vi "Inst.Krohn-Hite-7008.AppLauncher.vi"(8 "error in":errorcluster, 10 "Config Window":bool, 11 "Debug Mode":bool) -> (0 "error out":errorcluster)   [LabVIEW 2019, in "Inst.KH7008.lvlib" / "Inst.Krohn-Hite-7008.lvclass"]
uses:
  Inst.Krohn-Hite-7008.lvclass
  <vilib>/JKI/JKI SMO/SMO/SMO.lvclass
  <vilib>/JKI/JKI SMO/SMO/Typedefs/SMOState --Enum.ctl
  <vilib>/JKI/JKI SMO/SMO.UI/SMO.UI.lvclass
  <userlib>/LevyLab/Instrument Framework/Instrument UI/Instrument UI.lvclass
  Inst UI.Krohn-Hite-7008/Inst UI.Krohn-Hite-7008.lvclass
  <userlib>/LevyLab/Instrument Framework/Instrument/Instrument.lvclass
  C:/Program Files/National Instruments/LabVIEW 2019/vi.lib/JKI/JKI SMO/SMO/SMO.lvclass
  C:/Program Files/National Instruments/LabVIEW 2019/vi.lib/JKI/JKI SMO/SMO.UI/SMO.UI.lvclass
  C:/Program Files/National Instruments/LabVIEW 2019/user.lib/LevyLab/Instrument Framework/Instrument Types/Amplifier/Instrument.Amplifier.lvclass
  C:/Program Files/National Instruments/LabVIEW 2019/user.lib/LevyLab/Instrument Framework/Instrument/Instrument.lvclass
  C:/Program Files/National Instruments/LabVIEW 2019/user.lib/LevyLab/Instrument Framework/Instrument UI/Instrument UI.lvclass
panel:
  in  "Examine Configuration.ini":bool
  in  "Splash Status":string="Push Start to Start..." caption="String"
  in  "Start Application":bool caption="Play"
  in  "Stop Application":bool caption="Stop"
  out "UI SMO State":T1=enum."Stopped"
  out "SMO State":T1
  # "Example Instrument SMO Test Launcher"
  # "For instructions on how to use the JKI State Machine Objects, examples and video tutorials, visit:\nhttp://jki.net/state-machine-objects/\n\nJKI State Machine Objects™\nhttp://jki.net/state-machine-objects/\nCopyright (C) 2005-2015, JKI <info@jki.net>\nALL RIGHTS RESERVED"
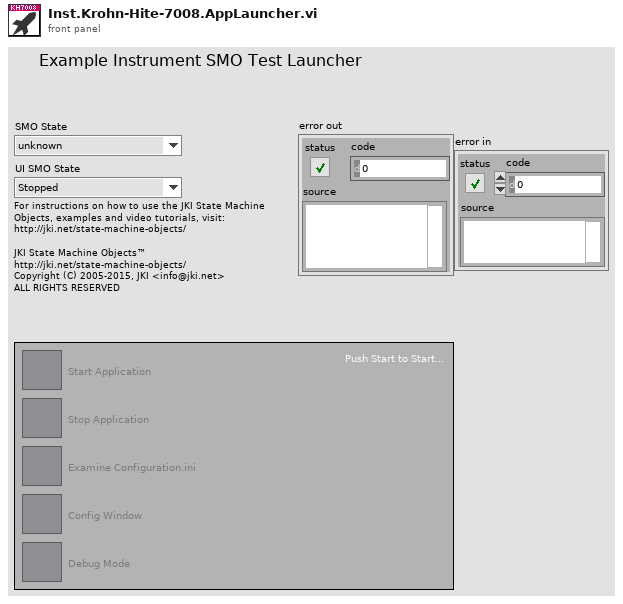
[diagram p1: front panel]
types:
  T1 = typedef "smo.lvlib/SMO.lvclass/SMOState --Enum.ctl" = enum16{"unknown", "Created", "Started", "Stopped"}
  T2 = enum32{"Invalid", "Standard", "Closed", "Hidden", "Minimized", "Maximized"}
  T3 = enum32{"invalid app kind", "Development System", "Run Time System", "Student Edition", "Embedded LabVIEW", "Evaluation", "Custom"}
  T4 = cluster{"Core":cluster{"Current VI Reference":refnum<vi>, "Close Panel on Exit?":bool}, "Instrument":refnum<class "Instrument.lvclass">, "Instrument UI":refnum<class "Instrument UI.lvclass">}
  T5 = cluster{"Current VI Reference":refnum<vi>, "Close Panel on Exit?":bool}
  T6 = typedef "smo.lvlib/SMO.lvclass/Public Events.ctl" = cluster{"Error":refnum<user-event>, "State":refnum<user-event>, "Reserve State":refnum<user-event>}
  T7 = cluster{"Event Registration Refnum":refnum<event-registration>, "Event Registration Refnum":refnum<event-registration>}
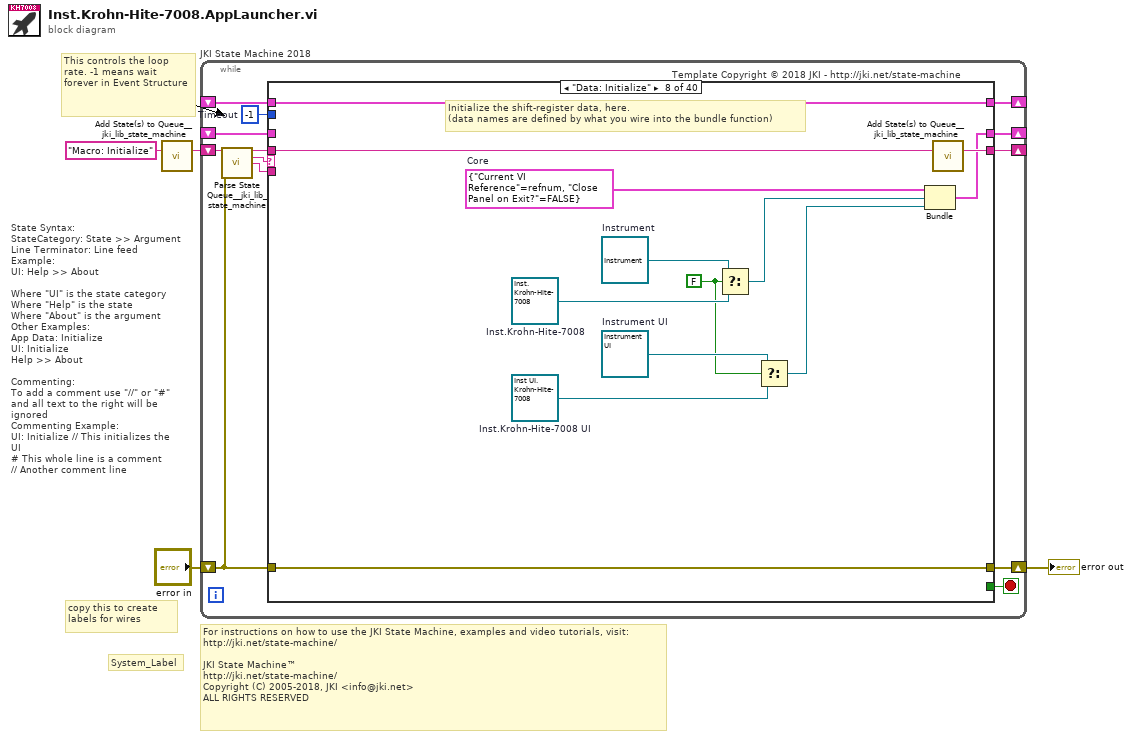
[diagram p0: block diagram]
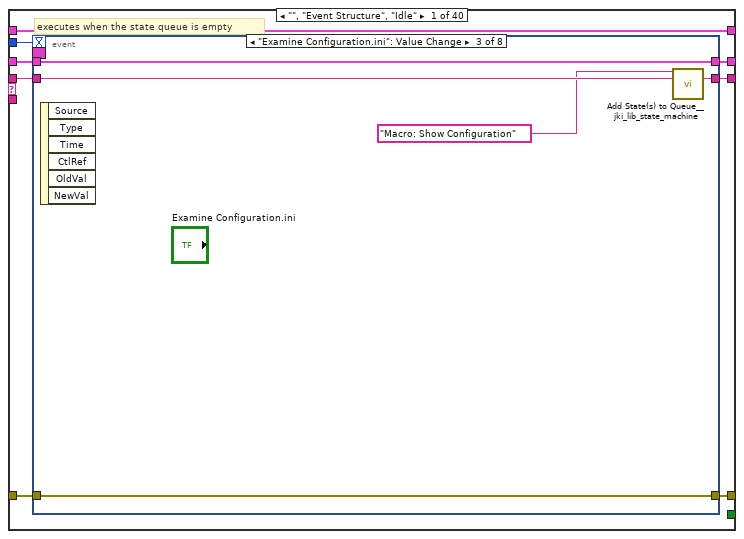
[diagram p2: hidden frame]
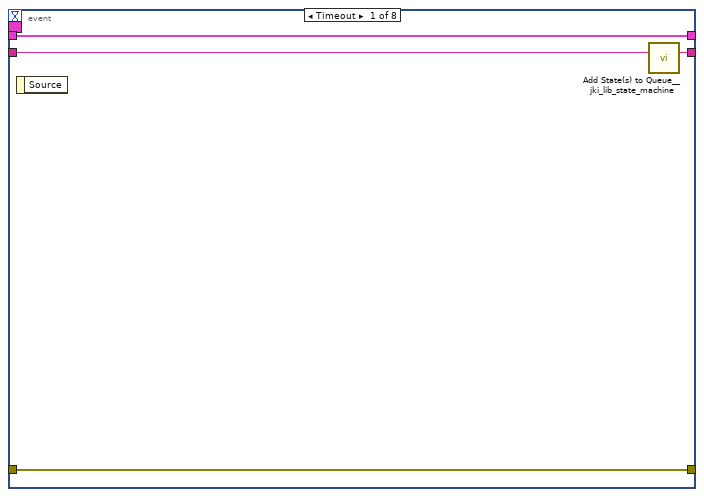
[diagram p3: hidden frame]
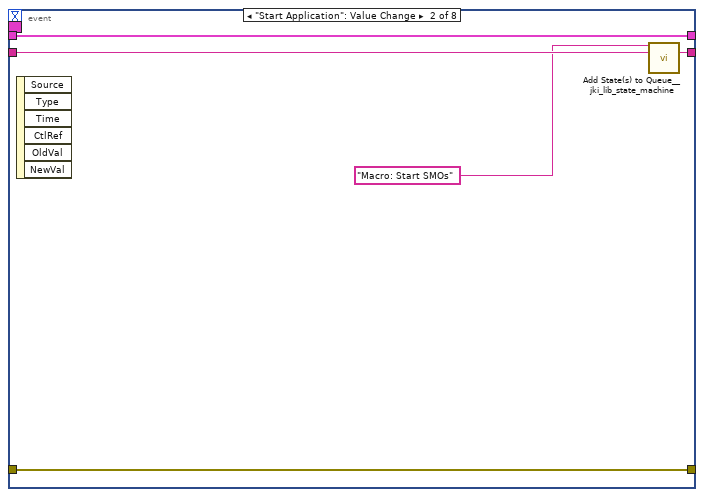
[diagram p4: hidden frame]
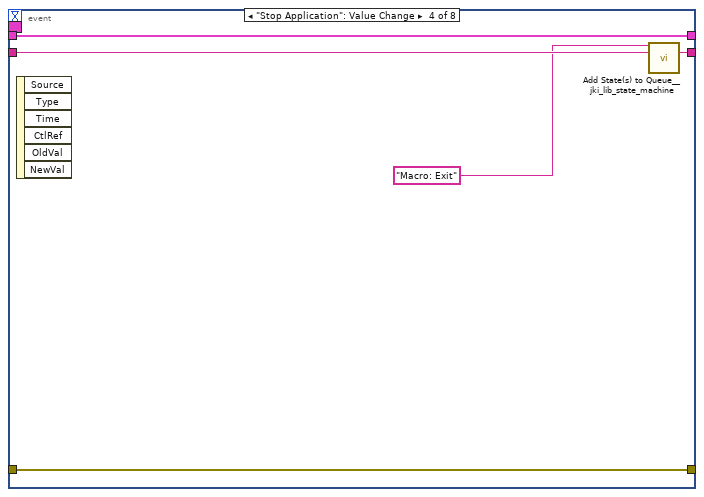
[diagram p5: hidden frame]
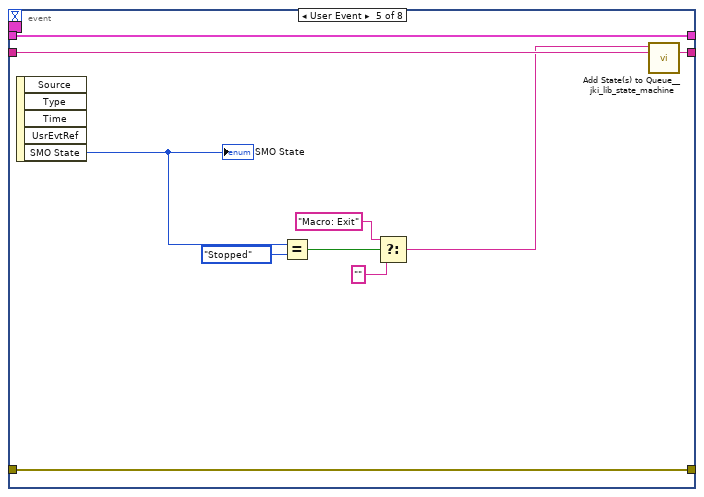
[diagram p6: hidden frame]
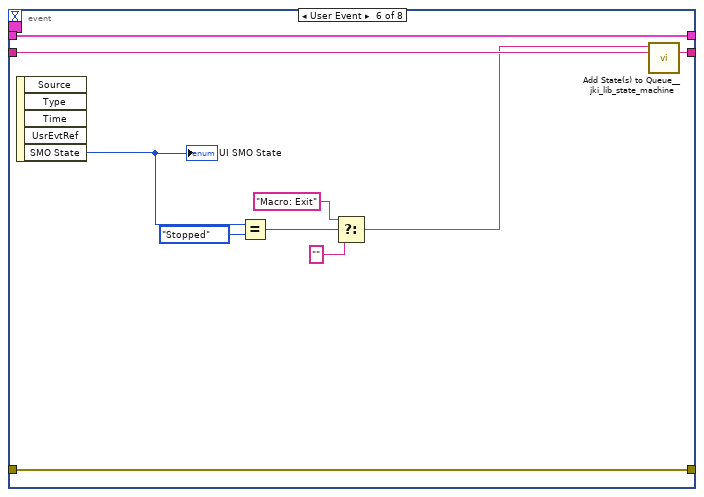
[diagram p7: hidden frame]
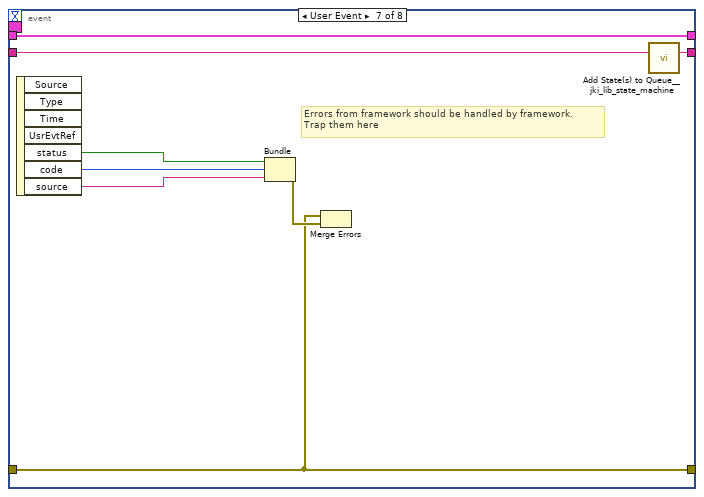
[diagram p8: hidden frame]
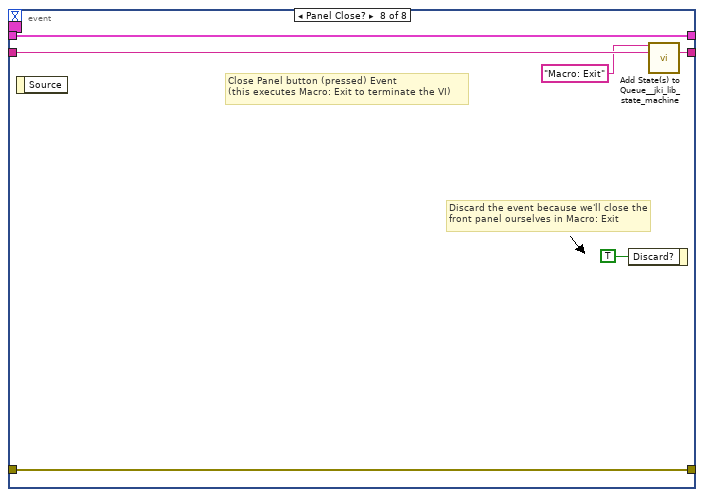
[diagram p9: hidden frame]
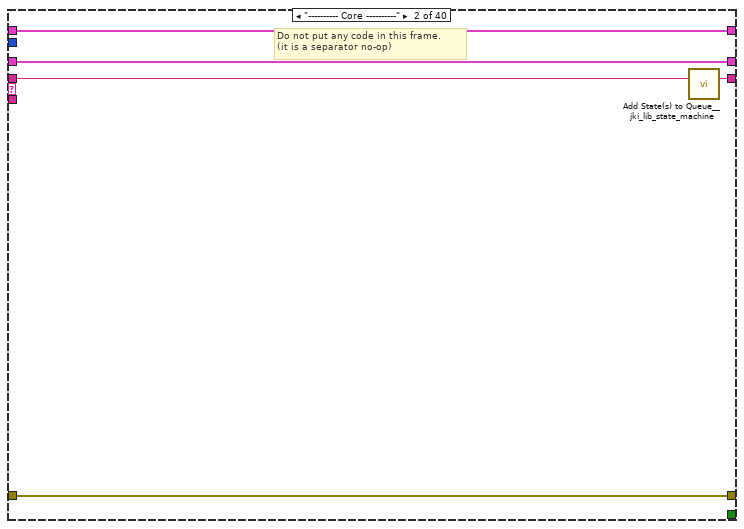
[diagram p10: hidden frame]
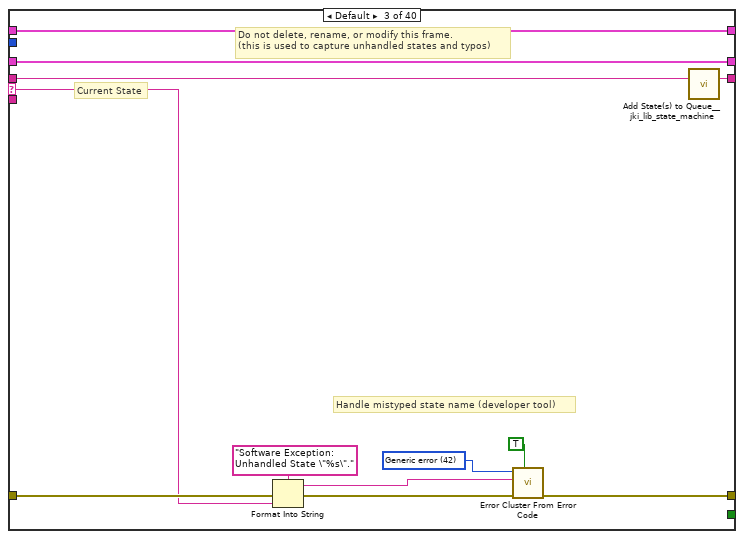
[diagram p11: hidden frame]
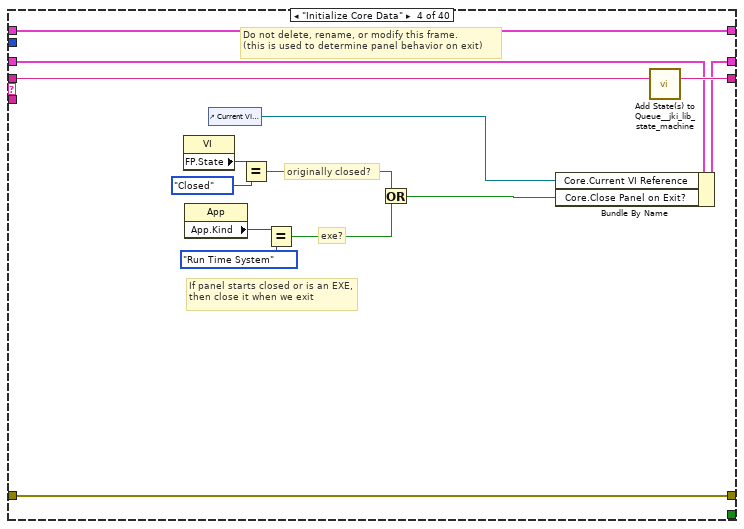
[diagram p12: hidden frame]
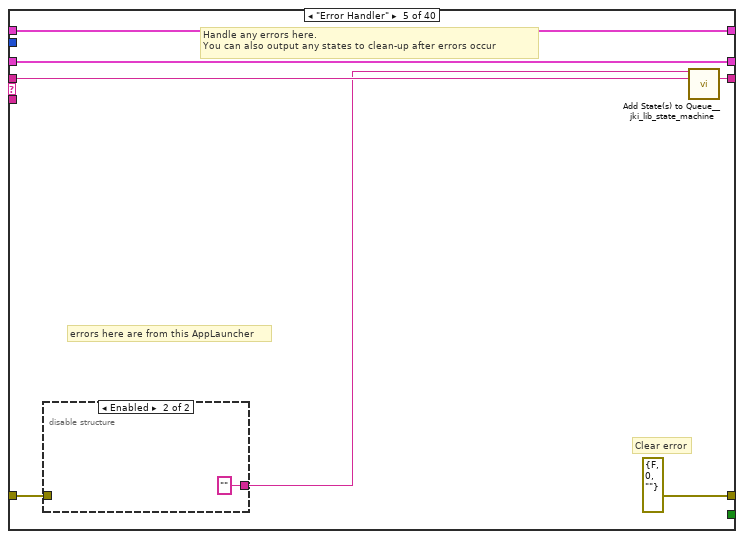
[diagram p13: hidden frame]
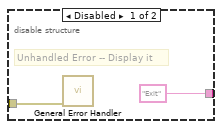
[diagram p14: hidden frame]
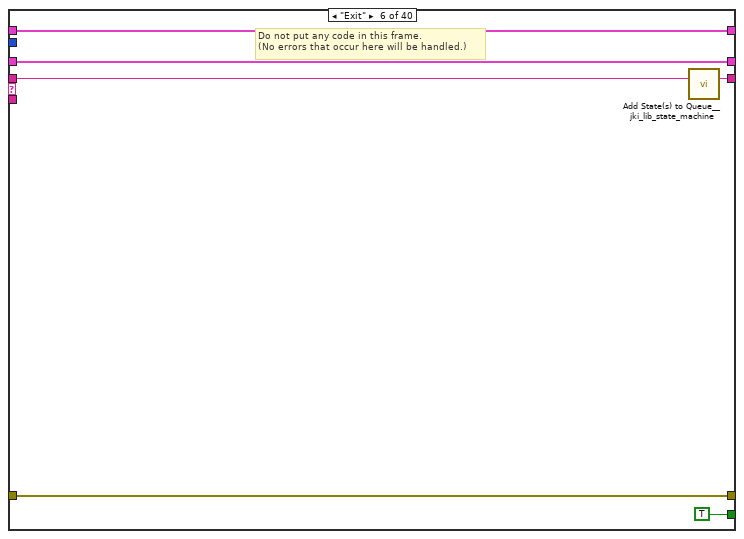
[diagram p15: hidden frame]
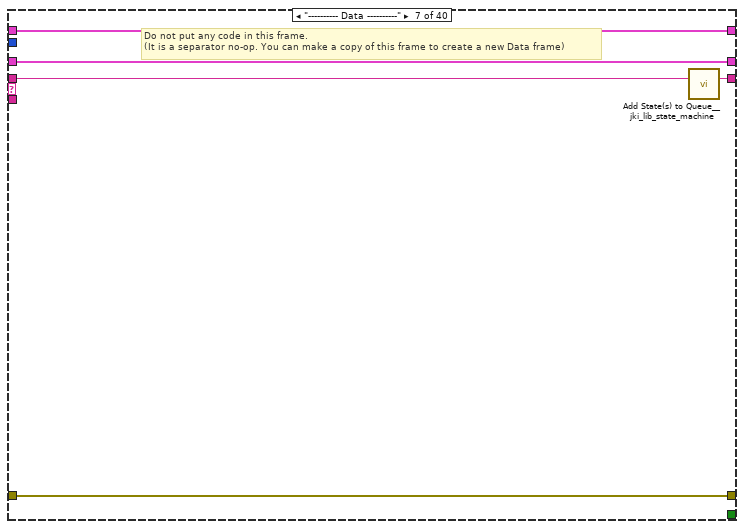
[diagram p16: hidden frame]
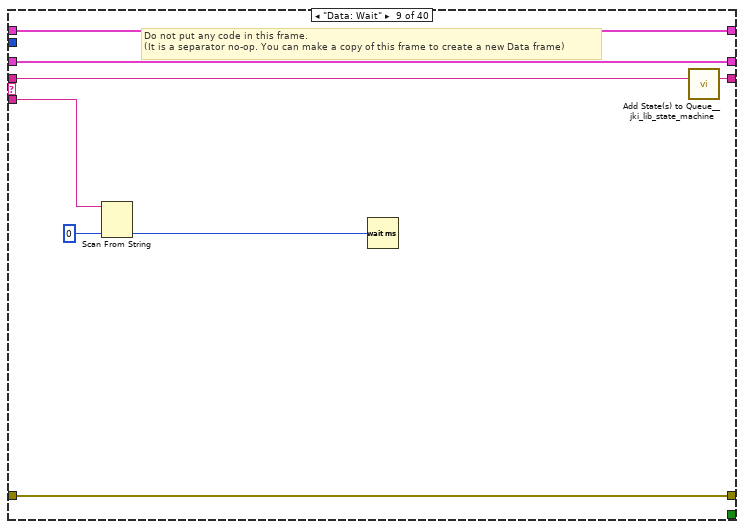
[diagram p17: hidden frame]
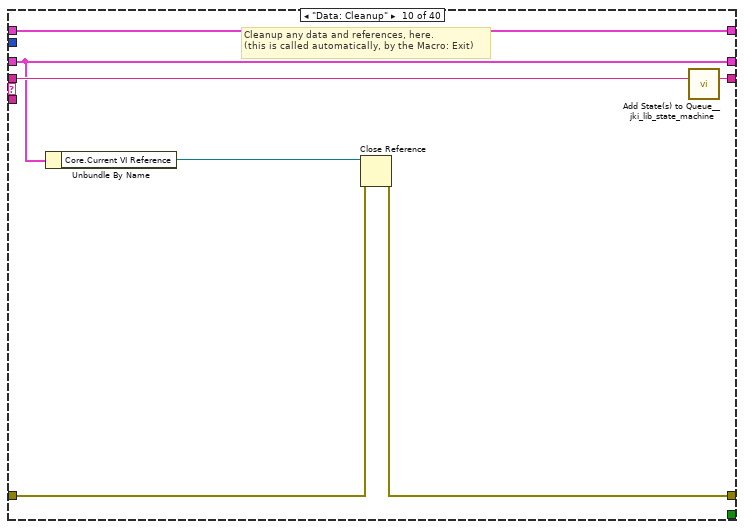
[diagram p18: hidden frame]
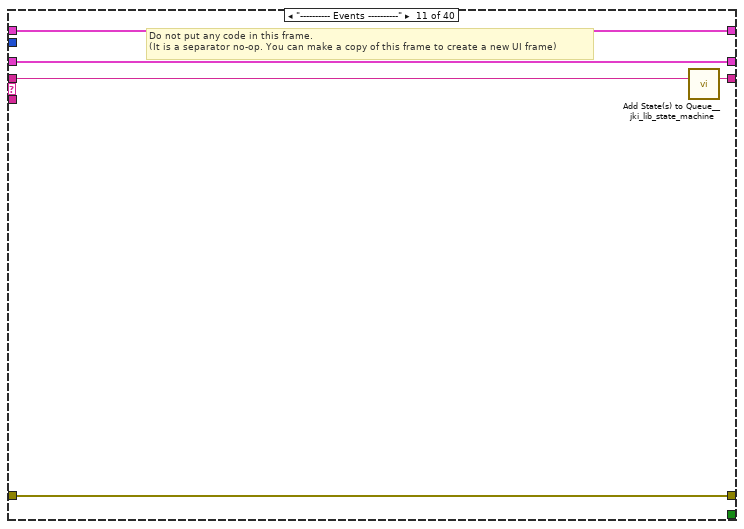
[diagram p19: hidden frame]
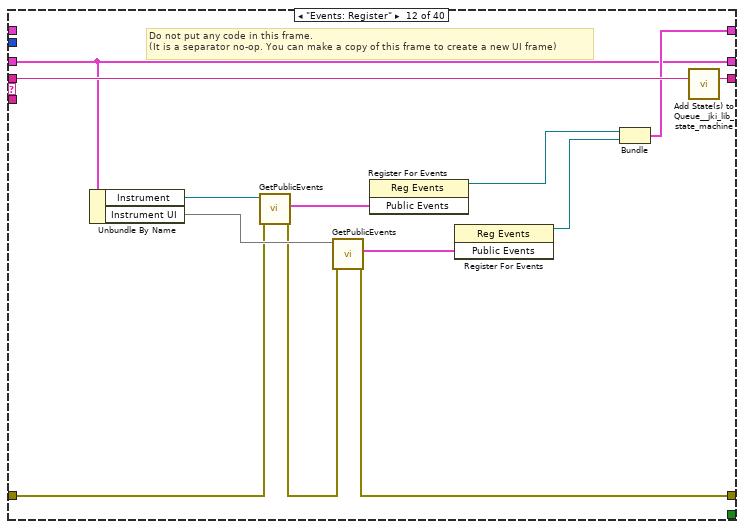
[diagram p20: hidden frame]
diagram:
  # "For instructions on how to use the JKI State Machine, examples and video tutorials, visit:\nhttp://jki.net/state-machine/\n\nJKI State Machine™\nhttp://jki.net/state-machine/\nCopyright (C) 2005-2018, JKI <info@jki.net>\nALL RIGHTS RESERVED"
  # "State Syntax:\nStateCategory: State >> Argument\nLine Terminator: Line feed\nExample:\nUI: Help >> About\n\nWhere \"UI\" is the state category\nWhere \"Help\" is the state\nWhere \"About\" is the argument\nOther Examples:\nApp Data: Initialize\nUI: Initialize\nHelp >> About\n\nCommenting:\nTo add a comment use \"//\" or \"#\" and all text to the right will be ignored\nCommenting Example:\nUI: Initialize // This initializes the UI\n# This whole line is a comment\n// Another comment line"
  # "copy this to create labels for wires"
  # "This controls the loop rate. -1 means wait forever in Event Structure"
  # "System_Label"
  n1 = call <vilib>:"Add State(s) to Queue__jki_lib_state_machine.vi"("State(s) in (\"\")"="Macro: Initialize") -> ("States Out"=w4:string)  [unwired: 14 in]
  n2 = while "JKI State Machine 2018" {
    shift-right: [w11] -> _
    shift-left: _ -> [w6]
    shift-right: [w14] -> w2
    shift-left: "error in" -> [w9]
    shift-right: [w13] -> _
    shift-left: w4 -> [w15]
    shift-right: [w8] -> _
    shift-left: _ -> [w7]
    stop <- w12 stop-if-true
    w10 = -1  # Timeout
    # "Template Copyright © 2018 JKI - http://jki.net/state-machine"
    n3 = call <vilib>:"Parse State Queue__jki_lib_state_machine.vi"("State Queue"=w15, "Error In (no error)"=w9) -> ("Remaining States"=w17:string, "Current State"=w5:string, "Arguments"=w16:string)  [unwired: 11 in]
    n4 = case shown="\"Data: Initialize\"" w5 {
      selector: w5 -> [_ _ w85 _ _ _ _ _ _ _ _ _ _ _ _ _ _ _ _ _ _ _ _ _ _ _ _ _ _ _ _ _ _ _ _ _ _ _ _ _]
      tunnel: w17 -> [w25 w83 w89 w109 w116 w125 w130 w143 w151 w158 w163 w176 w182 w187 w194 w201 w213 w291 w298 w303 w308 w314 w320 w326 w332 w344 w349 w360 w369 w379 w386 w397 w412 w427 w442 w457 w472 w481 w488 w493]
      tunnel: w16 -> [_ _ _ _ _ _ _ _ w146 _ _ _ _ _ _ w196 w207 _ _ _ _ _ _ _ _ _ _ _ _ _ _ _ _ _ _ _ _ _ w485 _]
      tunnel: [w22 w81 w91 w106 errorcluster {"status"=FALSE, "code"=0, "source"=""} ("error out") w122 w128 w138 w149 w154 w161 w165 w177 w185 w189 w197 w210 w281 w295 w301 w306 w312 w318 w324 w330 w342 w347 w356 w361 w370 w380 w393 w408 w423 w439 w454 w469 w479 w483 w491] -> w14
      tunnel: w9 -> [w21 w81 w90 w106 w112 w122 w128 w138 w149 w155 w161 w167 w178 w185 w191 w198 w211 w282 w292 w301 w306 w312 w318 w324 w330 w342 w347 w357 w362 w371 w381 w390 w404 w420 w437 w452 w465 w479 w484 w491]
      tunnel: [w24 w82 w88 w108 w115 w124 w129 w142 w150 w157 w162 w175 w181 w186 w193 w200 w212 w290 w297 w302 w307 w313 w319 w325 w331 w343 w348 w359 w368 w378 w385 w396 w411 w426 w441 w456 w471 w480 w487 w492] -> w13
      tunnel: [_ _ _ _ _ TRUE _ _ _ _ _ _ _ _ _ _ _ _ _ _ _ _ _ _ _ _ _ _ _ _ _ _ _ _ _ _ _ _ _ _] -> w12
      tunnel: [w20 w80 w87 w107 w113 w123 w127 w141 w148 w153 w160 w170 w180 w184 w192 w199 w209 w279 w294 w300 w305 w311 w317 w323 w329 w341 w346 w355 w364 w375 w383 w394 w409 w424 w438 w453 w468 w478 w486 w490] -> w11
      tunnel: w10 -> [w19 _ _ _ _ _ _ _ _ _ _ _ _ _ _ _ _ _ _ _ _ _ _ _ _ _ _ _ _ _ _ _ _ _ _ _ _ _ _ _]
      tunnel: [w18 w79 w84 w96 w111 w120 w126 w139 w147 w152 w159 w173 w179 w183 w190 w195 w206 w280 w296 w299 w304 w309 w315 w322 w328 w335 w345 w358 w367 w377 w384 w395 w410 w425 w440 w455 w470 w477 w482 w489] -> w8
      tunnel: w7 -> [w18 w79 w84 w96 w111 w120 w126 w139 w147 w152 w159 _ w179 w183 w190 w195 w206 w280 w296 w299 w304 w309 w315 w322 w328 w335 w345 w358 w367 w377 w384 w395 w410 w425 w440 w455 w470 w477 w482 w489]
      tunnel: w6 -> [w23 w80 w87 w102 w113 w123 w127 _ w148 w153 w160 w170 w180 w184 w192 w199 w209 w279 w294 w300 w305 w311 w317 w323 w329 w341 w346 w353 w365 w376 w383 w394 w409 w424 w438 w453 w468 w478 w486 w490]
      frame "", "Event Structure", "Idle" {
        # "executes when the state queue is empty"
        n5 = event shown="[2] \"Examine Configuration.ini\": Value Change" {
          selector: w18 -> [_ _ _ _ _ _ _ _]
          dyn-events: _ -> [_ _ _ _ _ _ _ _]
          timeout: w19 -> [_ _ _ _ _ _ _ _]
          tunnel: w25 -> [w29 w34 w39 w44 w54 w64 w72 w78]
          tunnel: [w28 w33 w38 w43 w53 w63 w71 w77] -> w24
          tunnel: w23 -> [w26 w31 w36 w41 w51 w61 w70 w75]
          tunnel: [w27 w32 w37 w42 w52 w62 w65 w76] -> w22
          tunnel: w21 -> [w27 w32 w37 w42 w52 w62 w65 w76]
          tunnel: [w26 w31 w36 w41 w51 w61 w70 w75] -> w20
          event Timeout {
            n6 = event-data() -> ()  [unwired: 1 in, 1 out]
            n7 = call <vilib>:"Add State(s) to Queue__jki_lib_state_machine.vi"("State(s) in (\"\")"=w29) -> ("States Out"=w28:string)  [unwired: 14 in]
          }
          event "Start Application": Value Change {
            n8 = event-data() -> ()  [unwired: 1 in, 6 out]
            n9 = call <vilib>:"Add State(s) to Queue__jki_lib_state_machine.vi"("State(s) in Front (\"\")"="Macro: Start SMOs" ("State(s) in Front (\"\")"), "State(s) in (\"\")"=w34) -> ("States Out"=w33:string)  [unwired: 13 in]
          }
          event "Examine Configuration.ini": Value Change {
            n10 = event-data() -> ()  [unwired: 1 in, 6 out]
            n11 = call <vilib>:"Add State(s) to Queue__jki_lib_state_machine.vi"("State(s) in Front (\"\")"="Macro: Show Configuration" ("State(s) in Front (\"\")"), "State(s) in (\"\")"=w39) -> ("States Out"=w38:string)  [unwired: 13 in]
          }
          event "Stop Application": Value Change {
            n12 = event-data() -> ()  [unwired: 1 in, 6 out]
            n13 = call <vilib>:"Add State(s) to Queue__jki_lib_state_machine.vi"("State(s) in Front (\"\")"="Macro: Exit" ("State(s) in Front (\"\")"), "State(s) in (\"\")"=w44) -> ("States Out"=w43:string)  [unwired: 13 in]
          }
          event User Event {
            n14 = event-data() -> ("SMO State"=w46:T1)  [unwired: 1 in, 4 out]
            "SMO State" <- w46
            n15 = Equal?(x=w46, y=SMOState_--Enum."Stopped") -> (x = y?=w49:bool)
            n16 = Select(t="Macro: Exit", s=w49, f="" ("State(s) in Front (\"\")")) -> (s? t:f=w45:string)
            n17 = call <vilib>:"Add State(s) to Queue__jki_lib_state_machine.vi"("State(s) in Front (\"\")"=w45, "State(s) in (\"\")"=w54) -> ("States Out"=w53:string)  [unwired: 13 in]
          }
          event User Event {
            n18 = event-data() -> ("SMO State"=w55:T1)  [unwired: 1 in, 4 out]
            "UI SMO State" <- w55
            n19 = Equal?(x=w55, y=SMOState_--Enum."Stopped") -> (x = y?=w59:bool)
            n20 = Select(t="Macro: Exit", s=w59, f="" ("State(s) in Front (\"\")")) -> (s? t:f=w57:string)
            n21 = call <vilib>:"Add State(s) to Queue__jki_lib_state_machine.vi"("State(s) in Front (\"\")"=w57, "State(s) in (\"\")"=w64) -> ("States Out"=w63:string)  [unwired: 13 in]
          }
          event User Event {
            # "Errors from framework should be handled by framework.\nTrap them here"
            n22 = event-data() -> ("status"=w66:bool, "code"=w68:i32, "source"=w67:string)  [unwired: 1 in, 4 out]
            n23 = Bundle("status"=w66, "code"=w68, "source"=w67) -> (w69:errorcluster)  [unwired: 1 in]
            n24 = Merge Errors(w65, w69) -> ()  [unwired: 1 out]
            n25 = call <vilib>:"Add State(s) to Queue__jki_lib_state_machine.vi"("State(s) in (\"\")"=w72) -> ("States Out"=w71:string)  [unwired: 14 in]
          }
          event Panel Close? {
            # "Discard the event because we'll close the front panel ourselves in Macro: Exit"
            # "Close Panel button (pressed) Event\n(this executes Macro: Exit to terminate the VI)"
            n26 = event-data() -> ()  [unwired: 1 in, 1 out]
            n27 = event-data("Discard?"=TRUE) -> ()  [unwired: 1 in, 1 out]
            n28 = call <vilib>:"Add State(s) to Queue__jki_lib_state_machine.vi"("State(s) in Front (\"\")"="Macro: Exit", "State(s) in (\"\")"=w78) -> ("States Out"=w77:string)  [unwired: 13 in]
          }
        }
      }
      frame "---------- Core ----------" {
        # "Do not put any code in this frame.\n(it is a separator no-op)"
        n29 = call <vilib>:"Add State(s) to Queue__jki_lib_state_machine.vi"("State(s) in (\"\")"=w83) -> ("States Out"=w82:string)  [unwired: 14 in]
      }
      frame Default {
        w94 = 42 items=["No error", "Argument error", "Memory is full", "Out of zone", "End of file", "File already open", "Generic file I/O error", "File not found", "File permission error", "Disk is full", "Duplicate path", "Too many files open", "System feature not enabled", "Resource file not found", "Cannot add resource", "Resource not found", "Image not found", "Image memory error", "Pen does not exist", "Config type invalid", "Config token not found", "Config parse error", "Config memory error", "Bad external code format", "Bad external code offset", "External code not present", "Null window", "Destroy window error", "Null menu", "Print aborted", "Bad print record", "Print driver error", "Windows error during printing", "Memory error during printing", "Print dialog error", "Generic print error", "Invalid device refnum", "Device not found", "Device parameter error", "Device unit error", "Cannot open device", "Device call aborted", "Generic error", "Cancelled by user", "Object ID too low", "Object ID too high", "Object not in heap", "Unknown heap", "Unknown object (invalid DefProc)", "Unknown object (DefProc not in table)", "Message out of range", "Invalid (null) method", "Unknown message", "Manager call not supported", "Bad address", "Network operation in progress", "Network operation timed out", "Connection is busy", "Network attribute not supported", "Network error", "Address in use", "System out of memory", "Connection aborted", "Connection refused", "Not connected", "Already connected", "Connection closed", "Initialization error (interapplication manager)", "Bad occurrence", "Wait on unbound occurrence handler", "Occurrence queue overflow", "Datalog type conflict", "Unused", "Unrecognized type (interapplication manager)", "Memory corrupt", "Failed to make temporary DLL", "Old CIN version", "Drag socket not found", "Failed to load drop-object", "Failed to register OLE object", "Failed to release OLE object", "Format specifier type mismatch", "Unknown format specifier", "Too few format specifiers", "Too many format specifiers", "Scan failed", "Newer CIN version", "Error converting to variant", "Runtime menu error", "Password tampered", "Variant attribute not found", "Incompatible variant data type", "Event data is not available", "Event Store is not present", "Occurrence is not found", "Event Queue is not created", "Event info is not available", "Refnum passed is NULL", "Error retrieving Class GUID", "Error retrieving CoClass GUID", "Error retrieving TypeLib GUID.", "Bad built application magic bytes.", "Specific driver is different from the specific driver associated with the Logical Name.", "There is no session opened to the class driver.", "Max Error", "MAX - Error with config objects", "MAX - Error loading configuration", "MAX - Group not supported"]
        # "Current State"
        # "Do not delete, rename, or modify this frame.\n(this is used to capture unhandled states and typos)"
        # "Handle mistyped state name (developer tool)"
        n30 = Format Into String(format string="Software Exception: Unhandled State \"%s\"." ("message"), error in=w90, w85) -> (resulting string=w93:string, error out=w92:errorcluster)  [unwired: 1 in]
        n31 = call <vilib>:"Error Cluster From Error Code.vi"("show call chain? (False)"=TRUE, "error in (no error)"=w92, "error message (\"\")"=w93, "error code (0)"=w94) -> ("error out"=w91:errorcluster)  [unwired: 5 in]
        n32 = call <vilib>:"Add State(s) to Queue__jki_lib_state_machine.vi"("State(s) in (\"\")"=w89) -> ("States Out"=w88:string)  [unwired: 14 in]
      }
      frame "Initialize Core Data" {
        # "Do not delete, rename, or modify this frame.\n(this is used to determine panel behavior on exit)"
        # "originally closed?"
        # "exe?"
        # "If panel starts closed or is an EXE, then close it when we exit"
        n33 = property class="VI"() -> ("FP.State"=w99:T2)  [unwired: 2 in, 2 out]
        n34 = property class="App"() -> ("App.Kind"=w105:T3)  [unwired: 2 in, 2 out]
        n35 = control-ref of="Current VI Reference"() -> (w100:refnum<vi>)
        n36 = Equal?(x=w99, y=T2."Closed" ("Front Panel Window:State")) -> (x = y?=w97:bool)
        n37 = Equal?(x=w105, y=T3."Run Time System" ("Application:Kind")) -> (x = y?=w103:bool)
        n38 = Or(x=w97, y=w103) -> (x .or. y?=w101:bool)
        n39 = Bundle By Name(cluster=w102, "Core.Current VI Reference"=w100, "Core.Close Panel on Exit?"=w101) -> (w107:T4)
        n40 = call <vilib>:"Add State(s) to Queue__jki_lib_state_machine.vi"("State(s) in (\"\")"=w109) -> ("States Out"=w108:string)  [unwired: 14 in]
      }
      frame "Error Handler" {
        # "errors here are from this AppLauncher"
        # "Handle any errors here.\nYou can also output any states to clean-up after errors occur"
        # "Clear error"
        n41 = disable-structure shown="Enabled" {
          disable-tunnel: w112 -> [w118 _]
          disable-tunnel: ["Exit" "" ("State(s) in Front (\"\")")] -> w110
          frame Disabled {
            # "Unhandled Error -- Display it"
            n42 = call <vilib>:"General Error Handler.vi"("error in (no error)"=w118) -> ()  [unwired: 10 in, 5 out]
          }
          frame Enabled {
          }
        }
        n43 = call <vilib>:"Add State(s) to Queue__jki_lib_state_machine.vi"("State(s) in Front (\"\")"=w110, "State(s) in (\"\")"=w116) -> ("States Out"=w115:string)  [unwired: 13 in]
      }
      frame "Exit" {
        # "Do not put any code in this frame.\n(No errors that occur here will be handled.)"
        n44 = call <vilib>:"Add State(s) to Queue__jki_lib_state_machine.vi"("State(s) in (\"\")"=w125) -> ("States Out"=w124:string)  [unwired: 14 in]
      }
      frame "---------- Data ----------" {
        # "Do not put any code in this frame.\n(It is a separator no-op. You can make a copy of this frame to create a new Data frame)"
        n45 = call <vilib>:"Add State(s) to Queue__jki_lib_state_machine.vi"("State(s) in (\"\")"=w130) -> ("States Out"=w129:string)  [unwired: 14 in]
      }
      frame "Data: Initialize" {
        w131 = FALSE ("s")
        w134 = refnum<class "Inst.Krohn-Hite-7008.lvclass"> refnum  # Inst.Krohn-Hite-7008
        w135 = refnum<class "Inst UI.Krohn-Hite-7008.lvclass"> refnum  # Inst.Krohn-Hite-7008 UI
        w136 = refnum<class "Instrument UI.lvclass"> refnum  # Instrument UI
        w137 = refnum<class "Instrument.lvclass"> refnum  # Instrument
        w140 = T5 {"Current VI Reference"=refnum, "Close Panel on Exit?"=FALSE}  # Core
        # "Initialize the shift-register data, here.\n(data names are defined by what you wire into the bundle function)"
        n46 = Select(t=w137, s=w131, f=w134) -> (s? t:f=w133:refnum<class "Instrument.lvclass">)
        n47 = Select(t=w136, s=w131, f=w135) -> (s? t:f=w132:refnum<class "Instrument UI.lvclass">)
        n48 = Bundle("Core"=w140, "Instrument"=w133, "Instrument UI"=w132) -> (w141:T4)  [unwired: 1 in]
        n49 = call <vilib>:"Add State(s) to Queue__jki_lib_state_machine.vi"("State(s) in (\"\")"=w143) -> ("States Out"=w142:string)  [unwired: 14 in]
      }
      frame "Data: Wait" {
        # "Do not put any code in this frame.\n(It is a separator no-op. You can make a copy of this frame to create a new Data frame)"
        n50 = Scan From String(input string=w146, default 1=u32 0) -> (output 1=w144:u32)  [unwired: 3 in, 3 out]
        n51 = Wait (ms)(milliseconds to wait=w144) -> ()  [unwired: 1 out]
        n52 = call <vilib>:"Add State(s) to Queue__jki_lib_state_machine.vi"("State(s) in (\"\")"=w151) -> ("States Out"=w150:string)  [unwired: 14 in]
      }
      frame "Data: Cleanup" {
        # "Cleanup any data and references, here.\n(this is called automatically, by the Macro: Exit)"
        n53 = Unbundle By Name(w153) -> ("Core.Current VI Reference"=w156:refnum<vi>)
        n54 = Close Reference(reference=w156, error in (no error)=w155) -> (error out=w154:errorcluster)
        n55 = call <vilib>:"Add State(s) to Queue__jki_lib_state_machine.vi"("State(s) in (\"\")"=w158) -> ("States Out"=w157:string)  [unwired: 14 in]
      }
      frame "---------- Events ----------" {
        # "Do not put any code in this frame.\n(It is a separator no-op. You can make a copy of this frame to create a new UI frame)"
        n56 = call <vilib>:"Add State(s) to Queue__jki_lib_state_machine.vi"("State(s) in (\"\")"=w163) -> ("States Out"=w162:string)  [unwired: 14 in]
      }
      frame "Events: Register" {
        # "Do not put any code in this frame.\n(It is a separator no-op. You can make a copy of this frame to create a new UI frame)"
        n57 = Unbundle By Name(w170) -> ("Instrument"=w169:refnum<class "Instrument.lvclass">, "Instrument UI"=w168)
        n58 = call <vilib>:"GetPublicEvents.vi"("error in (no error)"=w167, "SMO"=w169) -> ("error out"=w166:errorcluster, "Public Events"=w171:T6)  [unwired: 7 in, 1 out]
        n59 = call <vilib>:"GetPublicEvents.vi"("error in (no error)"=w166, "SMO"=w168) -> ("error out"=w165:errorcluster, "Public Events"=w172:T6)  [unwired: 7 in, 1 out]
        n60 = register-events(w171) -> (reference out=w174:refnum<event-registration>)  [unwired: 2 in, 1 out]
        n61 = register-events(w172) -> (reference out=w164:refnum<event-registration>)  [unwired: 2 in, 1 out]
        n62 = Bundle("Event Registration Refnum"=w174, "Event Registration Refnum"=w164) -> (w173:T7)  [unwired: 1 in]
        n63 = call <vilib>:"Add State(s) to Queue__jki_lib_state_machine.vi"("State(s) in (\"\")"=w176) -> ("States Out"=w175:string)  [unwired: 14 in]
      }
      frame "Events: Unregister" {
        # "Do not put any code in this frame.\n(It is a separator no-op. You can make a copy of this frame to create a new UI frame)"
        n64 = Unregister For Events(event registration refnum=w179, error in=w178) -> (error out=w177:errorcluster)
        n65 = call <vilib>:"Add State(s) to Queue__jki_lib_state_machine.vi"("State(s) in (\"\")"=w182) -> ("States Out"=w181:string)  [unwired: 14 in]
      }
      frame "---------- UI ----------" {
        # "Do not put any code in this frame.\n(It is a separator no-op. You can make a copy of this frame to create a new UI frame)"
        n66 = call <vilib>:"Add State(s) to Queue__jki_lib_state_machine.vi"("State(s) in (\"\")"=w187) -> ("States Out"=w186:string)  [unwired: 14 in]
      }
      frame "UI: Initialize" {
        # "Initialize the User Interface, here.\n(this is called automatically, by the Macro: Init)"
        n67 = invoke on="Stop Application" class="Bool" method="Reinit To Default"() -> ()  [unwired: 3 in, 3 out]
        n68 = invoke on="error out" class="Clust (strict)" method="Reinit To Default"() -> ()  [unwired: 3 in, 3 out]
        n69 = invoke on="SMO State 2" class="Enum (strict)" method="Reinit To Default"() -> ()  [unwired: 3 in, 3 out]
        n70 = invoke on="Start Application" class="Bool" method="Reinit To Default"() -> ()  [unwired: 3 in, 3 out]
        n71 = call <userlib>:"Fit VI window to Largest Dec__ogtk.vi"("error in (no error)"=w191, "border spacing (2 px)"=1) -> ("error out"=w189:errorcluster)  [unwired: 4 in, 1 out]
        n72 = call <vilib>:"Add State(s) to Queue__jki_lib_state_machine.vi"("State(s) in (\"\")"=w194) -> ("States Out"=w193:string)  [unwired: 14 in]
      }
      frame "UI: Cursor Set" {
        # "Argument"
        # "Set and Unset Cursor Busy.\n(Usage: \"UI: Cursor Set >> Busy|Idle\")"
        n73 = case shown="\"Busy\"" w196 {
          tunnel: w198 -> [w203 w205]
          tunnel: [w202 w204] -> w197
          frame "Idle", Default {
            n74 = call <vilib>:"Unset Busy.vi"("error in (no error)"=w203) -> ("error out"=w202:errorcluster)  [unwired: 10 in]
          }
          frame "Busy" {
            n75 = call <vilib>:"Set Busy.vi"("error in (no error)"=w205) -> ("error out"=w204:errorcluster)  [unwired: 9 in, 1 out]
          }
        }
        n76 = call <vilib>:"Add State(s) to Queue__jki_lib_state_machine.vi"("State(s) in (\"\")"=w201) -> ("States Out"=w200:string)  [unwired: 14 in]
      }
      frame "UI: Front Panel State" {
        # "Argument"
        # "Set Front Panel Open or Closed\n(Usage: \"UI: Front Panel State >> Open|Close\")"
        n77 = Unbundle By Name(w209) -> ("Core.Current VI Reference"=w208:refnum<vi>)
        n78 = case shown="\"Open\", \"Standard\", Default" w207 {
          tunnel: w211 -> [w219 w234 w245 w258 w271]
          tunnel: [w221 w235 w247 w260 w273] -> w210
          tunnel: w208 -> [w220 w232 w246 w259 w272]
          frame "Open", "Standard", Default {
            w214 = T2."Standard" ("State")
            n79 = property class="VI"(reference=w220, error in=w219) -> (reference out=w217:refnum<vi>, error out=w218:errorcluster, "FP.State"=w216:T2)
            n80 = Not Equal?(x=w216, y=w214) -> (x != y?=w215:bool)
            n81 = case shown="False" w215 {
              tunnel: [w225 w227] -> w221
              tunnel: w218 -> [w224 w227]
              tunnel: w217 -> [w223 _]
              tunnel: w214 -> [w222 _]
              frame True {
                n82 = invoke class="VI" method="FP.Open"(reference=w223, error in=w224, "Activate"=TRUE, "State"=w222) -> (error out=w225:errorcluster)  [unwired: 1 in, 4 out]
              }
              frame False {
              }
            }
          }
          frame "Close", "Closed" {
            n83 = property class="VI"(reference=w232, error in=w234) -> (reference out=w231:refnum<vi>, error out=w233:errorcluster, "FP.State"=w229:T2)
            n84 = Not Equal?(x=w229, y=T2."Closed" ("Front Panel Window:State")) -> (x != y?=w228:bool)
            n85 = case shown="True" w228 {
              tunnel: [w236 w239] -> w235
              tunnel: w233 -> [w236 w238]
              tunnel: w231 -> [_ w237]
              frame False {
              }
              frame True {
                n86 = invoke class="VI" method="FP.Close"(reference=w237, error in=w238) -> (error out=w239:errorcluster)  [unwired: 1 in, 2 out]
              }
            }
          }
          frame "Hidden", "Hide" {
            w240 = T2."Hidden" ("State")
            n87 = property class="VI"(reference=w246, error in=w245) -> (reference out=w243:refnum<vi>, error out=w244:errorcluster, "FP.State"=w242:T2)
            n88 = Not Equal?(x=w242, y=w240) -> (x != y?=w241:bool)
            n89 = case shown="True" w241 {
              tunnel: [w251 w252] -> w247
              tunnel: w244 -> [w250 w252]
              tunnel: w243 -> [w249 _]
              tunnel: w240 -> [w248 _]
              frame True {
                n90 = invoke class="VI" method="FP.Open"(reference=w249, error in=w250, "State"=w248) -> (error out=w251:errorcluster)  [unwired: 2 in, 4 out]
              }
              frame False {
              }
            }
          }
          frame "Minimize", "Minimized" {
            w253 = T2."Minimized" ("State")
            n91 = property class="VI"(reference=w259, error in=w258) -> (reference out=w256:refnum<vi>, error out=w257:errorcluster, "FP.State"=w255:T2)
            n92 = Not Equal?(x=w255, y=w253) -> (x != y?=w254:bool)
            n93 = case shown="True" w254 {
              tunnel: [w264 w265] -> w260
              tunnel: w257 -> [w263 w265]
              tunnel: w256 -> [w262 _]
              tunnel: w253 -> [w261 _]
              frame True {
                n94 = invoke class="VI" method="FP.Open"(reference=w262, error in=w263, "State"=w261) -> (error out=w264:errorcluster)  [unwired: 2 in, 4 out]
              }
              frame False {
              }
            }
          }
          frame "Maximize", "Maximized" {
            w266 = T2."Maximized" ("State")
            n95 = property class="VI"(reference=w272, error in=w271) -> (reference out=w269:refnum<vi>, error out=w270:errorcluster, "FP.State"=w268:T2)
            n96 = Not Equal?(x=w268, y=w266) -> (x != y?=w267:bool)
            n97 = case shown="True" w267 {
              tunnel: [w277 w278] -> w273
              tunnel: w270 -> [w276 w278]
              tunnel: w269 -> [w275 _]
              tunnel: w266 -> [w274 _]
              frame True {
                n98 = invoke class="VI" method="FP.Open"(reference=w275, error in=w276, "State"=w274) -> (error out=w277:errorcluster)  [unwired: 2 in, 4 out]
              }
              frame False {
              }
            }
          }
        }
        n99 = call <vilib>:"Add State(s) to Queue__jki_lib_state_machine.vi"("State(s) in (\"\")"=w213) -> ("States Out"=w212:string)  [unwired: 14 in]
      }
      frame "UI: Set Background Color" {
        # "Do not put any code in this frame.\n(It is a separator no-op. You can make a copy of this frame to create a new UI frame)"
        n100 = property class="VI"(error in=w282) -> (error out=w284:errorcluster, "Panel"=w285:refnum<vi>)  [unwired: 1 in, 1 out]
        n101 = property class="Pnl"(reference=w285, error in=w284) -> (error out=w283:errorcluster, "Panes[]"=w286:refnum<vi>[])  [unwired: 1 out]
        n102 = Index Array(array=w286, index=0) -> (element=w288:refnum<vi>)
        n103 = property class="Pane"(reference=w288, error in=w283, "PaneColor"=u32 16777238 ("Color Box")) -> (error out=w281:errorcluster)  [unwired: 1 out]
        n104 = call <vilib>:"Add State(s) to Queue__jki_lib_state_machine.vi"("State(s) in (\"\")"=w291) -> ("States Out"=w290:string)  [unwired: 14 in]
      }
      frame "UI: Open Configuration.ini" {
        # "Do not put any code in this frame.\n(It is a separator no-op. You can make a copy of this frame to create a new UI frame)"
        n105 = Unbundle By Name(w294) -> ("Instrument"=w293:refnum<class "Instrument.lvclass">)
        n106 = call <userlib>:"Examine Configuration.vi"("error in (no error)"=w292, "Instrument in"=w293) -> ("error out"=w295:errorcluster)  [unwired: 8 in, 1 out]
        n107 = call <vilib>:"Add State(s) to Queue__jki_lib_state_machine.vi"("State(s) in (\"\")"=w298) -> ("States Out"=w297:string)  [unwired: 14 in]
      }
      frame "UI: Exit" {
        # "Do not put any code in this frame.\n(It is a separator no-op. You can make a copy of this frame to create a new UI frame)"
        n108 = invoke on="Start Application" class="Bool" method="Reinit To Default"() -> ()  [unwired: 3 in, 3 out]
        n109 = invoke on="Stop Application" class="Bool" method="Reinit To Default"() -> ()  [unwired: 3 in, 3 out]
        n110 = call <vilib>:"Add State(s) to Queue__jki_lib_state_machine.vi"("State(s) in (\"\")"=w303) -> ("States Out"=w302:string)  [unwired: 14 in]
      }
      frame "---------- Macro ----------" {
        # "Do not put any code in this frame.\n(It is a separator no-op. You can make a copy of this frame to create a new Macro frame)"
        n111 = call <vilib>:"Add State(s) to Queue__jki_lib_state_machine.vi"("State(s) in (\"\")"=w308) -> ("States Out"=w307:string)  [unwired: 14 in]
      }
      frame "Macro: Initialize" {
        # "Initialization Macro\n(This is called once, when the VI starts)"
        n112 = call <vilib>:"Add State(s) to Queue__jki_lib_state_machine.vi"("State(s) in Front (\"\")"="Data: Initialize\nInitialize Core Data\n//Events: Register\nUI: Initialize\nUI: Front Panel State >> Open\nUI: Set Background Color\nSplash: Set Status >> ...", "State(s) in (\"\")"=w314) -> ("States Out"=w313:string)  [unwired: 13 in]
      }
      frame "Macro: Show Configuration" {
        # "Initialization Macro\n(This is called once, when the VI starts)"
        n113 = call <vilib>:"Add State(s) to Queue__jki_lib_state_machine.vi"("State(s) in Front (\"\")"="Splash: Set Status >> Opeing Configuration...\nUI: Open Configuration.ini\nData: Wait >> 1000\nSplash: Set Status >> ...", "State(s) in (\"\")"=w320) -> ("States Out"=w319:string)  [unwired: 13 in]
      }
      frame "Macro: Start SMOs" {
        # "Do not put any code in this frame.\n(It is a separator no-op. You can make a copy of this frame to create a new Macro frame)"
        n114 = call <vilib>:"Add State(s) to Queue__jki_lib_state_machine.vi"("State(s) in Front (\"\")"="Splash: Set Status >> Creating Instrument...\nSMO: Create Instrument\nData: Wait >> 100\nSplash: Set Status >> Creating Instrument UI...\nSMO: Create Instrument UI\nData: Wait >> 100\nSplash: Set Status >> Registering Events...\nEvents: Register\nData: Wait >> 100\nSplash: Set Status >> Starting Instrument...\nSMO: Start Instrument\nData: Wait >> 100\nSplash: Set Status >> Instrument Process Started...\nData: Wait >> 100\nSplash: Set Status >> Starting User Interface...\nSMO: Start Instrument UI\nData: Wait >> 100\nUI: Front Panel State >> Hide\nSMO: Show Instrument UI" ("State(s) in Front (\"\")"), "State(s) in (\"\")"=w326) -> ("States Out"=w325:string)  [unwired: 13 in]
      }
      frame "Macro: Stop SMOs" {
        # "#todo\nshould stopping UI go before stopping Instrument?"
        # "Do not put any code in this frame.\n(It is a separator no-op. You can make a copy of this frame to create a new Macro frame)"
        n115 = call <vilib>:"Add State(s) to Queue__jki_lib_state_machine.vi"("State(s) in Front (\"\")"="UI: Front Panel State >> Show\nSplash: Set Status >> Stopping Instrument...\nSMO: Stop Instrument\nData: Wait >> 100\nSplash: Set Status >> Destroying Instrument...\nSMO: Destroy Instrument\nData: Wait >> 100\nSplash: Set Status >>Hiding UI...\nSMO: Hide Instrument UI\nData: Wait >> 100\nSplash: Set Status >> Stopping UI...\nSMO: Stop Instrument UI\nData: Wait >> 100\nSplash: Set Status >> Destroying UI...\nSMO: Destroy Instrument UI" ("State(s) in Front (\"\")"), "State(s) in (\"\")"=w332) -> ("States Out"=w331:string)  [unwired: 13 in]
      }
      frame "Macro: Exit" {
        # "Exit Macro\n(This is called once, when the VI exits)"
        n116 = Unbundle By Name(w341) -> ("Core.Close Panel on Exit?"=w340:bool)
        n117 = Select(t="UI: Front Panel State >> Close", s=w340, f="" ("Empty String Constant")) -> (s? t:f=w337:string)
        n118 = call <vilib>:"Add State(s) to Queue__jki_lib_state_machine.vi"("State(s) in Front (\"\")"="UI: Front Panel State >> Open\nUI: Exit\nMacro: Stop SMOs", "State(s) in (\"\")"=w337, "State(s) at Back (\"\")"="Data: Cleanup\nEvents: Unregister\nExit") -> ("States Out"=w336:string)  [unwired: 12 in]
        n119 = call <vilib>:"Add State(s) to Queue__jki_lib_state_machine.vi"("State(s) in Front (\"\")"=w336, "State(s) in (\"\")"=w344) -> ("States Out"=w343:string)  [unwired: 13 in]
      }
      frame "---------- SMO ----------" {
        # "Do not put any code in this frame.\n(It is a separator no-op. You can make a copy of this frame to create a new Macro frame)"
        n120 = call <vilib>:"Add State(s) to Queue__jki_lib_state_machine.vi"("State(s) in (\"\")"=w349) -> ("States Out"=w348:string)  [unwired: 14 in]
      }
      frame "SMO: Create Instrument" {
        # "Do not put any code in this frame.\n(It is a separator no-op. You can make a copy of this frame to create a new Macro frame)"
        n121 = Unbundle By Name(w353) -> ("Instrument"=w352:refnum<class "Instrument.lvclass">)
        n122 = call <userlib>:"Create Instrument SMO.vi"("error in (no error)"=w357, "Debug Mode? [F]"="Debug Mode", "Configuration Window? [T]"="Config Window", "Instrument in"=w352) -> ("error out"=w356:errorcluster, "Instrument out"=w354:refnum<class "Instrument.lvclass">)  [unwired: 6 in]
        n123 = Bundle By Name(cluster=w353, "Instrument"=w354) -> (w355:T4)
        n124 = call <vilib>:"Add State(s) to Queue__jki_lib_state_machine.vi"("State(s) in (\"\")"=w360) -> ("States Out"=w359:string)  [unwired: 14 in]
      }
      frame "SMO: Start Instrument" {
        # "Do not put any code in this frame.\n(It is a separator no-op. You can make a copy of this frame to create a new Macro frame)"
        n125 = Unbundle By Name(w365) -> ("Instrument"=w366:refnum<class "Instrument.lvclass">)
        n126 = call <vilib>:"Start.vi"("error in (no error)"=w362, "SMO"=w366) -> ("error out"=w361:errorcluster, "SMO out"=w363:refnum<class "Instrument.lvclass">)  [unwired: 8 in]
        n127 = Bundle By Name(cluster=w365, "Instrument"=w363) -> (w364:T4)
        n128 = call <vilib>:"Add State(s) to Queue__jki_lib_state_machine.vi"("State(s) in (\"\")"=w369) -> ("States Out"=w368:string)  [unwired: 14 in]
      }
      frame "SMO: Create Instrument UI" {
        # "Do not put any code in this frame.\n(It is a separator no-op. You can make a copy of this frame to create a new Macro frame)"
        n129 = Unbundle By Name(w376) -> ("Instrument UI"=w374:refnum<class "Instrument UI.lvclass">, "Instrument"=w373:refnum<class "Instrument.lvclass">)
        n130 = call <userlib>:"Create UI.vi"("error in (no error)"=w371, "Instrument in"=w373, "Instrument UI"=w374) -> ("error out"=w370:errorcluster, "Instrument UI out"=w372:refnum<class "Instrument UI.lvclass">)  [unwired: 7 in]
        n131 = Bundle By Name(cluster=w376, "Instrument UI"=w372) -> (w375:T4)
        n132 = call <vilib>:"Add State(s) to Queue__jki_lib_state_machine.vi"("State(s) in (\"\")"=w379) -> ("States Out"=w378:string)  [unwired: 14 in]
      }
      frame "SMO: Start Instrument UI" {
        # "Do not put any code in this frame.\n(It is a separator no-op. You can make a copy of this frame to create a new Macro frame)"
        n133 = Unbundle By Name(w383) -> ("Instrument UI"=w382:refnum<class "Instrument UI.lvclass">)
        n134 = call <vilib>:"Start.vi"("error in (no error)"=w381, "SMO"=w382) -> ("error out"=w380:errorcluster)  [unwired: 8 in, 1 out]
        n135 = call <vilib>:"Add State(s) to Queue__jki_lib_state_machine.vi"("State(s) in (\"\")"=w386) -> ("States Out"=w385:string)  [unwired: 14 in]
      }
      frame "SMO: Show Instrument UI" {
        # "Do not put any code in this frame.\n(It is a separator no-op. You can make a copy of this frame to create a new Macro frame)"
        n136 = Unbundle By Name(w394) -> ("Instrument UI"=w392:refnum<class "Instrument UI.lvclass">)
        n137 = call <vilib>:"GetState.vi"("error in (no error)"=w390, "SMO"=w392) -> ("error out"=w388:errorcluster, "SMO State"=w387:T1, "SMO out"=w391:refnum<class "Instrument UI.lvclass">)  [unwired: 7 in]
        n138 = call <vilib>:"Clear Errors.vi"("error in (no error)"=w388) -> ("error out"=w389:errorcluster)  [unwired: 5 in, 1 out]
        n139 = case shown="\"Started\"" w387 {
          tunnel: [w398 w401] -> w393
          tunnel: w391 -> [_ w400]
          tunnel: w389 -> [w398 w399]
          frame Default {
          }
          frame "Started" {
            n140 = call <vilib>:"Show.vi"("error in (no error)"=w399, "SMO.UI"=w400) -> ("error out"=w401:errorcluster)  [unwired: 8 in, 1 out]
          }
        }
        n141 = call <vilib>:"Add State(s) to Queue__jki_lib_state_machine.vi"("State(s) in (\"\")"=w397) -> ("States Out"=w396:string)  [unwired: 14 in]
      }
      frame "SMO: Destroy Instrument" {
        # "Do not put any code in this frame.\n(It is a separator no-op. You can make a copy of this frame to create a new Macro frame)"
        n142 = Unbundle By Name(w409) -> ("Instrument"=w407:refnum<class "Instrument.lvclass">)
        n143 = call <vilib>:"GetState.vi"("error in (no error)"=w404, "SMO"=w407) -> ("error out"=w403:errorcluster, "SMO State"=w406:T1, "SMO out"=w402:refnum<class "Instrument.lvclass">)  [unwired: 7 in]
        n144 = call <vilib>:"Clear Errors.vi"("error in (no error)"=w403) -> ("error out"=w405:errorcluster)  [unwired: 5 in, 1 out]
        n145 = case shown="\"Stopped\"" w406 {
          tunnel: [w413 w416] -> w408
          tunnel: w405 -> [w413 w415]
          tunnel: w402 -> [_ w414]
          frame Default {
          }
          frame "Stopped" {
            n146 = call <vilib>:"Destroy.vi"("error in (no error)"=w415, "SMO"=w414) -> ("error out"=w416:errorcluster)  [unwired: 9 in]
          }
        }
        n147 = call <vilib>:"Add State(s) to Queue__jki_lib_state_machine.vi"("State(s) in (\"\")"=w412) -> ("States Out"=w411:string)  [unwired: 14 in]
      }
      frame "SMO: Hide Instrument UI" {
        # "Do not put any code in this frame.\n(It is a separator no-op. You can make a copy of this frame to create a new Macro frame)"
        n148 = Unbundle By Name(w424) -> ("Instrument UI"=w422:refnum<class "Instrument UI.lvclass">)
        n149 = call <vilib>:"GetState.vi"("error in (no error)"=w420, "SMO"=w422) -> ("error out"=w418:errorcluster, "SMO State"=w417:T1, "SMO out"=w421:refnum<class "Instrument UI.lvclass">)  [unwired: 7 in]
        n150 = call <vilib>:"Clear Errors.vi"("error in (no error)"=w418) -> ("error out"=w419:errorcluster)  [unwired: 5 in, 1 out]
        n151 = case shown="Default" w417 {
          tunnel: [w428 w431] -> w423
          tunnel: w421 -> [_ w430]
          tunnel: w419 -> [w428 w429]
          frame Default {
          }
          frame "Started" {
            n152 = call <vilib>:"Hide.vi"("error in (no error)"=w429, "SMO.UI"=w430) -> ("error out"=w431:errorcluster)  [unwired: 8 in, 1 out]
          }
        }
        n153 = call <vilib>:"Add State(s) to Queue__jki_lib_state_machine.vi"("State(s) in (\"\")"=w427) -> ("States Out"=w426:string)  [unwired: 14 in]
      }
      frame "SMO: Stop Instrument UI" {
        # "Do not put any code in this frame.\n(It is a separator no-op. You can make a copy of this frame to create a new Macro frame)"
        n154 = Unbundle By Name(w438) -> ("Instrument UI"=w433:refnum<class "Instrument UI.lvclass">)
        n155 = call <vilib>:"GetState.vi"("error in (no error)"=w437, "SMO"=w433) -> ("error out"=w436:errorcluster, "SMO State"=w434:T1, "SMO out"=w432:refnum<class "Instrument UI.lvclass">)  [unwired: 7 in]
        n156 = call <vilib>:"Clear Errors.vi"("error in (no error)"=w436) -> ("error out"=w435:errorcluster)  [unwired: 5 in, 1 out]
        n157 = case shown="\"Created\", \"Started\"" w434 {
          tunnel: [w443 w446] -> w439
          tunnel: w432 -> [_ w445]
          tunnel: w435 -> [w443 w444]
          frame Default {
          }
          frame "Created", "Started" {
            n158 = call <vilib>:"Stop.vi"("error in (no error)"=w444, "SMO"=w445) -> ("error out"=w446:errorcluster)  [unwired: 8 in, 1 out]
          }
        }
        n159 = call <vilib>:"Add State(s) to Queue__jki_lib_state_machine.vi"("State(s) in (\"\")"=w442) -> ("States Out"=w441:string)  [unwired: 14 in]
      }
      frame "SMO: Stop Instrument" {
        # "Do not put any code in this frame.\n(It is a separator no-op. You can make a copy of this frame to create a new Macro frame)"
        n160 = Unbundle By Name(w453) -> ("Instrument"=w448:refnum<class "Instrument.lvclass">)
        n161 = call <vilib>:"GetState.vi"("error in (no error)"=w452, "SMO"=w448) -> ("error out"=w451:errorcluster, "SMO State"=w449:T1, "SMO out"=w447:refnum<class "Instrument.lvclass">)  [unwired: 7 in]
        n162 = call <vilib>:"Clear Errors.vi"("error in (no error)"=w451) -> ("error out"=w450:errorcluster)  [unwired: 5 in, 1 out]
        n163 = case shown="\"Created\", \"Started\"" w449 {
          tunnel: [w458 w461] -> w454
          tunnel: w447 -> [_ w460]
          tunnel: w450 -> [w458 w459]
          frame Default {
          }
          frame "Created", "Started" {
            n164 = call <vilib>:"Stop.vi"("error in (no error)"=w459, "SMO"=w460) -> ("error out"=w461:errorcluster)  [unwired: 8 in, 1 out]
          }
        }
        n165 = call <vilib>:"Add State(s) to Queue__jki_lib_state_machine.vi"("State(s) in (\"\")"=w457) -> ("States Out"=w456:string)  [unwired: 14 in]
      }
      frame "SMO: Destroy Instrument UI" {
        # "Do not put any code in this frame.\n(It is a separator no-op. You can make a copy of this frame to create a new Macro frame)"
        n166 = Unbundle By Name(w468) -> ("Instrument UI"=w467:refnum<class "Instrument UI.lvclass">)
        n167 = call <vilib>:"GetState.vi"("error in (no error)"=w465, "SMO"=w467) -> ("error out"=w464:errorcluster, "SMO State"=w462:T1, "SMO out"=w466:refnum<class "Instrument UI.lvclass">)  [unwired: 7 in]
        n168 = call <vilib>:"Clear Errors.vi"("error in (no error)"=w464) -> ("error out"=w463:errorcluster)  [unwired: 5 in, 1 out]
        n169 = case shown="Default" w462 {
          tunnel: w463 -> [w473 w476]
          tunnel: [w473 w475] -> w469
          tunnel: w466 -> [_ w474]
          frame Default {
          }
          frame "Stopped" {
            n170 = call <vilib>:"Destroy.vi"("error in (no error)"=w476, "SMO"=w474) -> ("error out"=w475:errorcluster)  [unwired: 9 in]
          }
        }
        n171 = call <vilib>:"Add State(s) to Queue__jki_lib_state_machine.vi"("State(s) in (\"\")"=w472) -> ("States Out"=w471:string)  [unwired: 14 in]
      }
      frame "---------- Splash ----------" {
        # "Template Separator\n(You can make a copy of, or modify, this frame)"
        n172 = call <vilib>:"Add State(s) to Queue__jki_lib_state_machine.vi"("State(s) in (\"\")"=w481) -> ("States Out"=w480:string)  [unwired: 14 in]
      }
      frame "Splash: Set Status" {
        # "Your code here.\n(You can make a copy of, or modify, this frame)"
        n173 = property on="Splash Status" class="Str"(error in=w484, "Value"=w485) -> (error out=w483:errorcluster)  [unwired: 1 in, 1 out]
        n174 = call <vilib>:"Add State(s) to Queue__jki_lib_state_machine.vi"("State(s) in (\"\")"=w488) -> ("States Out"=w487:string)  [unwired: 14 in]
      }
      frame "Splash: 2" {
        # "Your code here.\n(You can make a copy of, or modify, this frame)"
        n175 = call <vilib>:"Add State(s) to Queue__jki_lib_state_machine.vi"("State(s) in (\"\")"=w493) -> ("States Out"=w492:string)  [unwired: 14 in]
      }
    }
  }
  "error out" <- w2
